vi "Event Structure 1.vi"() -> ()   [LabVIEW 2020]
panel:
  out "Value":i32
  in  "Stop":bool
  in  "Boolean":bool
  # "Event Structure"
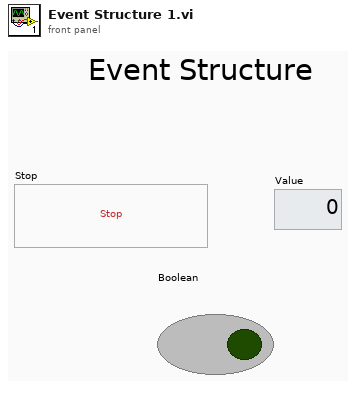
[diagram p1: front panel]
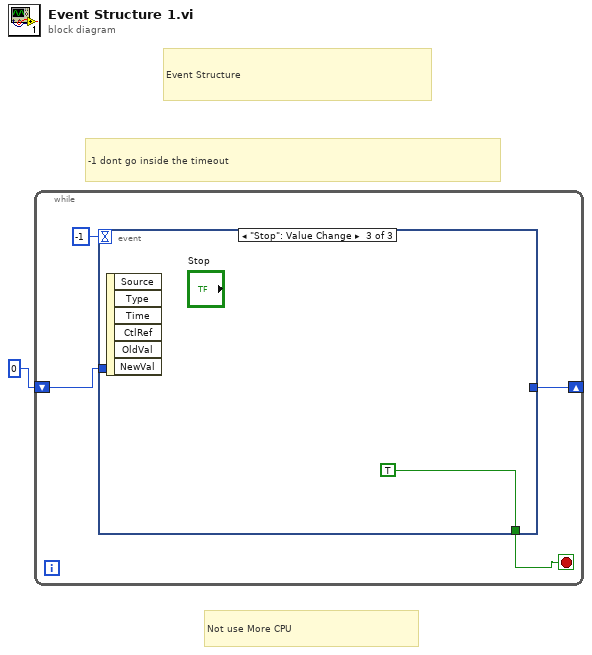
[diagram p0: block diagram]
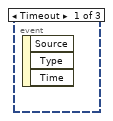
[diagram p2: hidden frame]
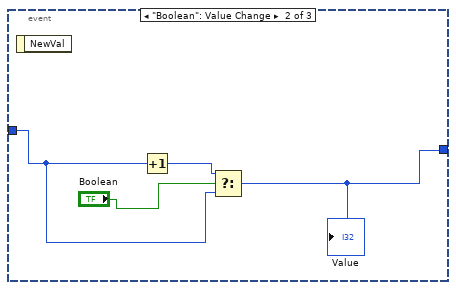
[diagram p3: hidden frame]
diagram:
  # "Not use More CPU"
  # "-1 dont go inside the timeout"
  # "Event Structure"
  n1 = while {
    shift-right: [w4] -> _
    shift-left: 0 -> [w5]
    stop <- w2 stop-if-true
    n2 = event shown="[2] \"Stop\": Value Change" {
      selector: _ -> [_ _ _]
      dyn-events: _ -> [_ _ _]
      timeout: -1 -> [_ _ _]
      tunnel: w5 -> [_ w6 _]
      tunnel: [_ w8 _] -> w4
      tunnel: [_ _ TRUE] -> w2
      event Timeout {
        n3 = event-data() -> ()  [unwired: 1 in, 3 out]
      }
      event "Boolean": Value Change {
        n4 = event-data() -> ()  [unwired: 1 in, 1 out]
        n5 = Increment(x=w6) -> (x+1=w9:i32)
        n6 = Select(t=w9, s="Boolean", f=w6) -> (s? t:f=w8:i32)
        "Value" <- w8
      }
      event "Stop": Value Change {
        n7 = event-data() -> ()  [unwired: 1 in, 6 out]
      }
    }
  }
